vi "Test comms.vi"() -> ()   [LabVIEW 2016]
uses:
  Actuator/Controls/Command list.ctl
  Actuator/Controls/Command cluster.ctl
  <vilib>/Instr/_visa.llb/VISA Configure Serial Port (Instr).vi
panel:
  out "resulting string":string
  out "Array":string[](array[string])
  in  "Cancel Button":bool
  out "Numeric 2":dbl
  out "String 2":string
  in  "Displacement 2":dbl format="%#_13g"
  out "output 1":u16
  in  "Enum":T1=enum."£ncal"
  out "read string 3":string
  out "x-y":u32
  out "read string 2":string
  in  "Displacement":dbl format="%#_13g"
  in  "stop":bool
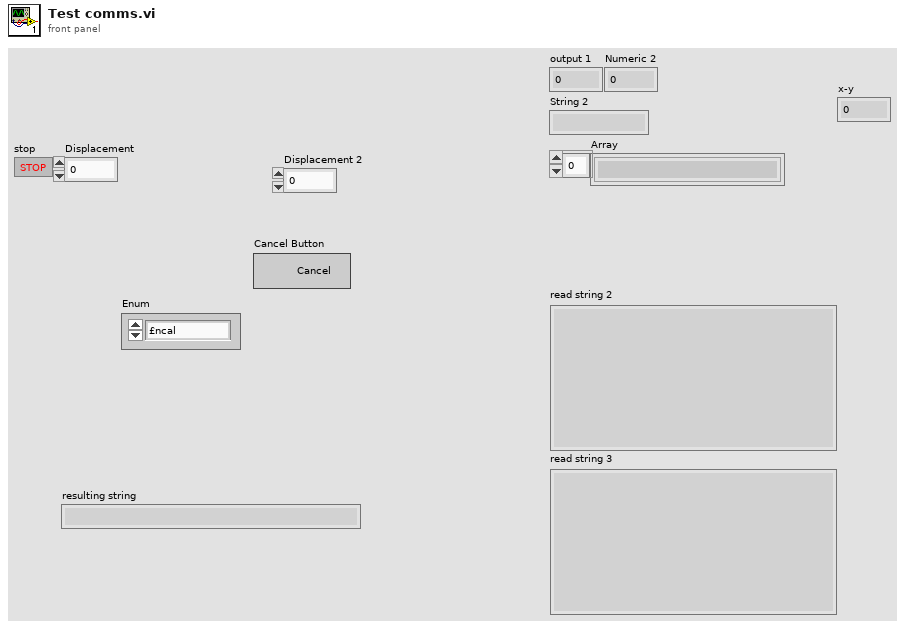
[diagram p1: front panel]
types:
  T1 = typedef "Command list.ctl" = enum16{"", "£nabort", "getaxisno", "£getserialno", "£nidentify", "&&£setnlimit", "&£nm", "&£snv", "&£speed", "£np", "£ncal"}
  T2 = typedef "Command cluster.ctl" = cluster{"Command":T1, "data":variant}
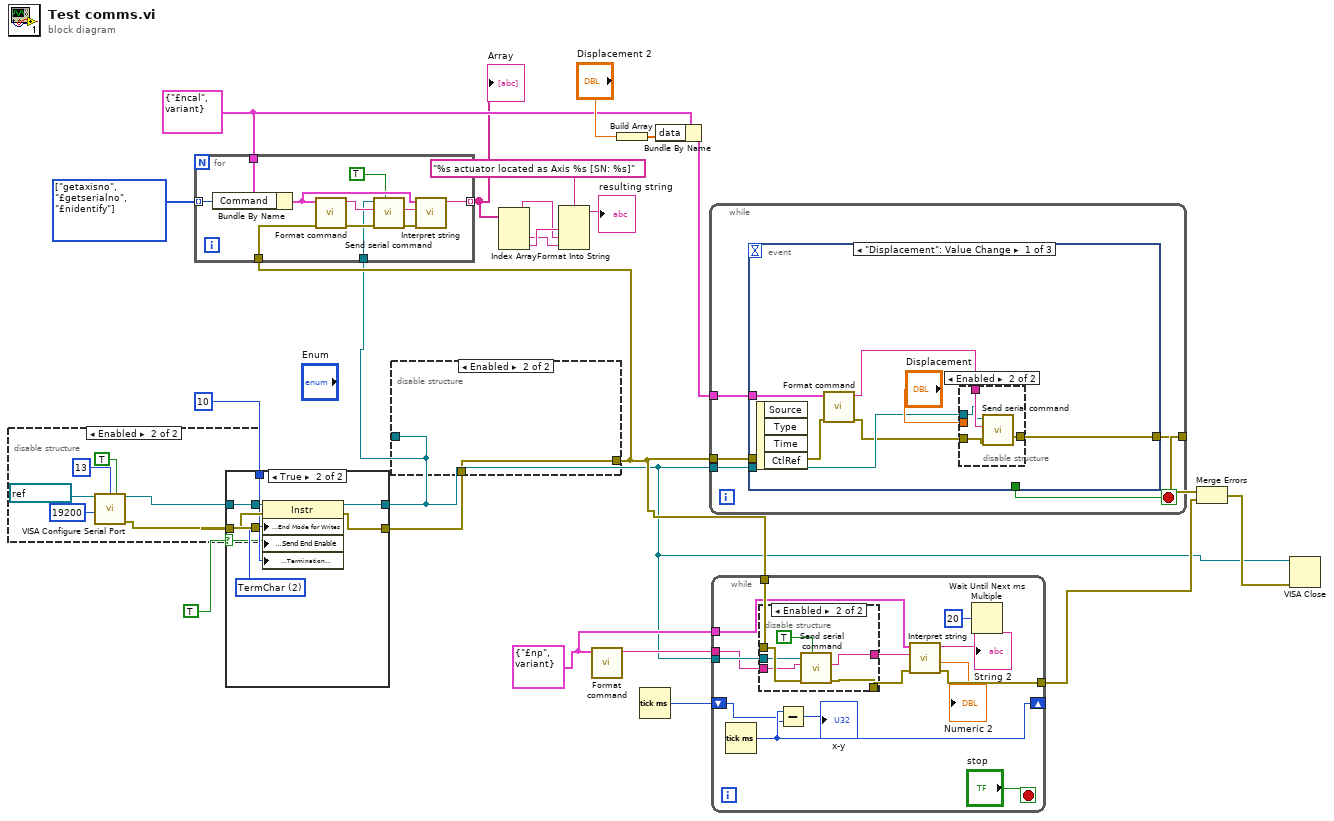
[diagram p0: block diagram]
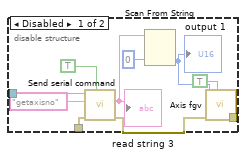
[diagram p2: hidden frame]
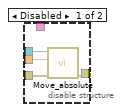
[diagram p3: hidden frame]
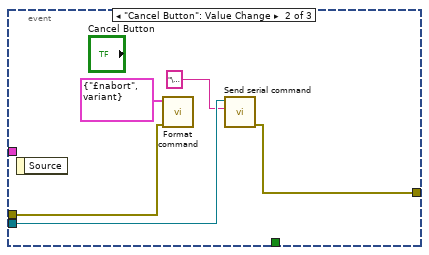
[diagram p4: hidden frame]
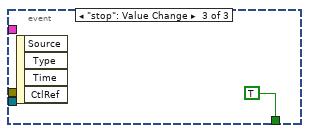
[diagram p5: hidden frame]
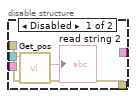
[diagram p6: hidden frame]
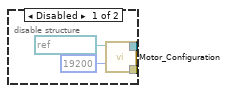
[diagram p8: hidden frame]
diagram:
  w9 = T1[] [enum."getaxisno", enum."£getserialno", enum."£nidentify"] items=["", "£nabort", "getaxisno", "£getserialno", "£nidentify", "&&£setnlimit", "&£nm", "&£snv", "&£speed", "£np", "£ncal"]
  w10 = T2 {"Command"=enum."£ncal", "data"=variant} ("Cluster")
  w11 = T2 {"Command"=enum."£np", "data"=variant} ("Cluster")
  n1 = disable-structure shown="Enabled" {
    disable-tunnel: [w26 w32] -> w22
    disable-tunnel: [w25 w31] -> w23
    frame Disabled {
      n2 = call "Motor_Configuration.vi"("baud rate"=u32 19200, "VISA resource name"=refnum<visa-resource-name> "COM4") -> ("error out"=w26:errorcluster, "reference out"=w25:refnum<visa-resource-name>)  [unwired: 8 in]
    }
    frame Enabled {
      n3 = call-poly "VISA Configure Serial Port"("VISA resource name"=refnum<visa-resource-name> "COM4", "termination char\n(0xA = '\\n' = LF)"=u8 13 ("termination char\n(0xA = '\\n' = LF)"), "Enable Termination\nChar (T)"=TRUE ("Enable Termination\nChar (T)"), "baud rate (9600)"=u32 19200) -> ("VISA resource name out"=w31:refnum<visa-resource-name>, "error out"=w32:errorcluster)  [unwired: 6 in, 4 out]
    }
  }
  n4 = case shown="True" TRUE {
    selector: TRUE -> [_ w38]
    tunnel: w23 -> [w35 w43]
    tunnel: w22 -> [w36 w42]
    tunnel: [w35 w41] -> w7
    tunnel: [w36 w37] -> w16
    tunnel: u8 10 ("termination char\n(0xA = '\\n' = LF)") -> [_ w39]
    frame False {
    }
    frame True {
      w40 = u16 2 items=["None", "LastBit", "TermChar", "Break"] ("Serial Settings:Serial End Mode for Writes")
      n5 = property class="Instr"(reference=w43, error in=w42, "Serial Settings:End Mode for Writes"=w40, "Message Based Settings:Send End Enable"=w38, "Message Based Settings:Termination Character"=w39) -> (reference out=w41:refnum<visa-resource-name>, error out=w37:errorcluster)
    }
  }
  n6 = disable-structure shown="Enabled" {
    disable-tunnel: w16 -> [w51 w54]
    disable-tunnel: [w45 w54] -> w8
    disable-tunnel: w7 -> [w44 _]
    frame Disabled {
      n7 = call "Send serial command.vi"("Read?"=TRUE, "error IO"=w51, "Send string"="getaxisno", "VISA resource name out"=w44) -> ("error out"=w46:errorcluster, "read string"=w50:string)  [unwired: 5 in, 1 out]
      "read string 3" <- w50
      n8 = Scan From String(input string=w50, default 1=u16 0) -> (output 1=w48:u16)  [unwired: 3 in, 3 out]
      "output 1" <- w48
      n9 = call "Axis fgv.vi"("Set"=TRUE, "error in (no error)"=w46, "Axis"=w48) -> ("error out"=w45:errorcluster)  [unwired: 7 in, 1 out]
    }
    frame Enabled {
    }
  }
  n10 = for {
    tunnel: w10 -> [w65]
    tunnel: w9 -> [w64] mode=indexing
    tunnel: w8 -> [w63]
    tunnel: w7 -> [w60]
    tunnel: [w55] -> w6 mode=indexing
    n11 = Bundle By Name(cluster=w65, "Command"=w64) -> (w59:T2)
    n12 = call "Format command.vi"("error in (no error)"=w63, "Cluster"=w59) -> ("error out"=w62:errorcluster, "String"=w61:string)  [unwired: 8 in]
    n13 = call "Send serial command.vi"("Read?"=TRUE, "error IO"=w62, "Send string"=w61, "VISA resource name out"=w60) -> ("error out"=w57:errorcluster, "read string"=w58:string)  [unwired: 5 in, 1 out]
    n14 = call "Interpret string.vi"("error in (no error)"=w57, "String"=w58, "Cluster"=w59) -> ("String 2"=w55:string)  [unwired: 5 in, 3 out]
  }
  "Array" <- w6
  n15 = Index Array(array=w6) -> (element #1=w2:string, element #2=w1:string, element #3=w3:string)  [unwired: 3 in]
  n16 = Format Into String(format string="%s actuator located as Axis %s [SN: %s]", w3, w2, w1) -> (resulting string=→"resulting string":string)  [unwired: 2 in, 1 out]
  n17 = call "Format command.vi"("Cluster"=w11) -> ("String"=w12:string)  [unwired: 9 in, 1 out]
  n18 = Build Array("Displacement 2") -> (w14:dbl[])
  n19 = Tick Count (ms)() -> (millisecond timer value=w17:u32)
  n20 = Bundle By Name(cluster=w10, "data"=w14) -> (w13:T2)
  n21 = while {
    tunnel: w7 -> [w70]
    tunnel: w8 -> [w69]
    tunnel: [w67] -> w20
    tunnel: w13 -> [w66]
    stop <- w68 stop-if-true
    n22 = event shown="[0] \"Displacement\": Value Change" {
      selector: _ -> [_ _ _]
      dyn-events: _ -> [_ _ _]
      timeout: _ -> [_ _ _]
      tunnel: w70 -> [w76 w88 _]
      tunnel: w69 -> [w74 w89 _]
      tunnel: [_ _ TRUE] -> w68
      tunnel: [w75 w87 _] -> w67
      tunnel: w66 -> [w72 _ _]
      event "Displacement": Value Change {
        n23 = event-data() -> ()  [unwired: 1 in, 4 out]
        n24 = call "Format command.vi"("error in (no error)"=w74, "Cluster"=w72) -> ("error out"=w73:errorcluster, "String"=w71:string)  [unwired: 8 in]
        n25 = disable-structure shown="Enabled" {
          disable-tunnel: "Displacement" -> [w81 _]
          disable-tunnel: w76 -> [w80 w84]
          disable-tunnel: [w79 w82] -> w75
          disable-tunnel: w73 -> [w78 w83]
          disable-tunnel: w71 -> [_ w85]
          frame Disabled {
            n26 = call "Move_absolute.vi"("error IO"=w78, "Displacement"=w81, "VISA resource name"=w80) -> ("error out"=w79:errorcluster)  [unwired: 7 in, 1 out]
          }
          frame Enabled {
            n27 = call "Send serial command.vi"("error IO"=w83, "Send string"=w85, "VISA resource name out"=w84) -> ("error out"=w82:errorcluster)  [unwired: 6 in, 2 out]
          }
        }
      }
      event "Cancel Button": Value Change {
        n28 = event-data() -> ()  [unwired: 1 in, 1 out]
        n29 = call "Format command.vi"("error in (no error)"=w89, "Cluster"=T2 {"Command"=enum."£nabort", "data"=variant} ("Cluster 2")) -> ()  [unwired: 8 in, 2 out]
        n30 = call "Send serial command.vi"("Send string"="\u0003", "VISA resource name out"=w88) -> ("error out"=w87:errorcluster)  [unwired: 7 in, 2 out]
      }
      event "stop": Value Change {
        n31 = event-data() -> ()  [unwired: 1 in, 4 out]
      }
    }
  }
  n32 = while {
    tunnel: w8 -> [w103]
    tunnel: w7 -> [w102]
    tunnel: [w94] -> w19
    shift-right: [w101] -> _
    shift-left: w17 -> [w100]
    tunnel: w12 -> [w98]
    tunnel: w11 -> [w96]
    stop <- "stop" stop-if-true
    n33 = Tick Count (ms)() -> (millisecond timer value=w101:u32)
    n34 = disable-structure shown="Enabled" {
      disable-tunnel: w103 -> [w109 w115]
      disable-tunnel: w102 -> [w108 w114]
      disable-tunnel: [w107 w111] -> w97
      disable-tunnel: w98 -> [_ w113]
      disable-tunnel: [_ w110] -> w95
      frame Disabled {
        n35 = call "Get_pos.vi"("error IO"=w109, "VISA resource name out"=w108) -> ("error out"=w107:errorcluster, "read string"=→"read string 2":string)  [unwired: 7 in, 1 out]
      }
      frame Enabled {
        n36 = call "Send serial command.vi"("Read?"=TRUE, "error IO"=w115, "Send string"=w113, "VISA resource name out"=w114) -> ("error out"=w111:errorcluster, "read string"=w110:string)  [unwired: 5 in, 1 out]
      }
    }
    n37 = Subtract(x=w101, y=w100) -> (x-y=→"x-y":u32)
    n38 = call "Interpret string.vi"("error in (no error)"=w97, "String"=w95, "Cluster"=w96) -> ("error out"=w94:errorcluster, "Numeric 2"=→"Numeric 2":dbl, "String 2"=→"String 2":string)  [unwired: 5 in, 1 out]
    n39 = Wait Until Next ms Multiple(millisecond multiple=u32 20) -> ()  [unwired: 1 out]
  }
  n40 = Merge Errors(w20, w19) -> (w18:errorcluster)
  n41 = VISA Close(VISA resource name=w7, error in (no error)=w18) -> ()  [unwired: 1 out]
